vi "Query_Temp_Path.vi"(8 "error in (no error)":errorcluster, 11 "Dest_NI_MSIPath in":refnum<class "Dest_NI_MSIPath.lvclass">) -> (0 "error out":errorcluster, 3 "Dest_NI_MSIPath out":refnum<class "Dest_NI_MSIPath.lvclass">)   [LabVIEW 2020, in "Dest_NI_MSIPath.lvclass"]
uses:
  <vilib>/AppBuilder/IB_Classes/Dest_NI_MSIPath/Dest_NI_MSIPath.lvclass
  <vilib>/AppBuilder/IB_Classes/Dest_NI_MSIPath/Dest_NI_MSIPath.lvclass/Dest_NI_MSIPath.ctl
  kernel32.dll
  <vilib>/AppBuilder/IB_Classes/Destination/niLabel/niLabel.lvclass
  e:/builds/penguin/labview/branches/2020/dev/dist/vi.lib/AppBuilder/IB_Classes/Destination/niLabel/niLabel.lvclass
  e:/builds/penguin/labview/branches/2020/dev/dist/vi.lib/AppBuilder/IB_Classes/Destination/IB_Destination.lvclass
  e:/builds/penguin/labview/branches/2020/dev/dist/vi.lib/AppBuilder/IB_Classes/Dest_NI_MSIPath/Dest_NI_MSIPath.lvclass
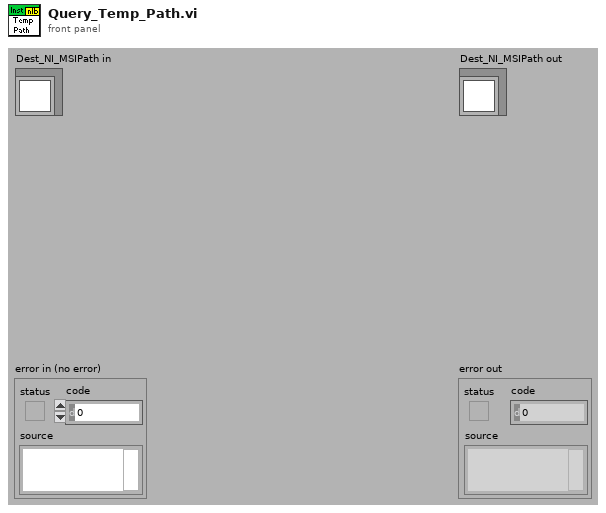
[diagram p1: front panel]
types:
  T1 = typedef "IB_Dest_niLabel.ctl" = cluster{"local path":path}
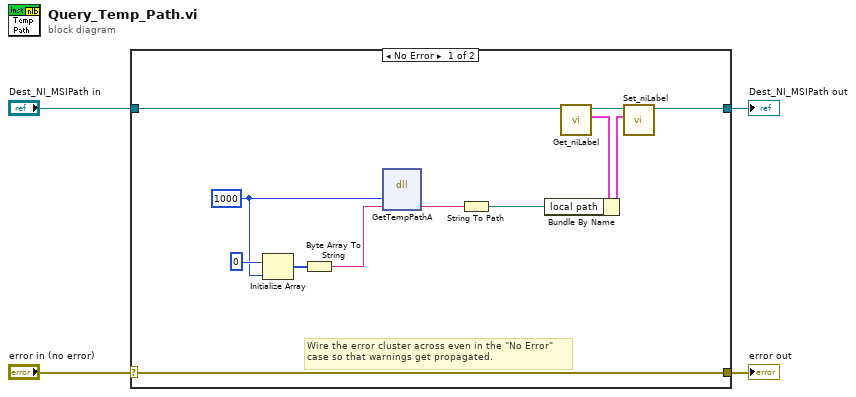
[diagram p0: block diagram]
diagram:
  n1 = case shown="No Error" "error in (no error)" {
    selector: "error in (no error)" -> [w16 w18]
    tunnel: [w16 w18] -> w3
    tunnel: [w7 w17] -> w1
    tunnel: "Dest_NI_MSIPath in" -> [w6 w17]
    frame No Error {
      w11 = u32 1000 ("dimension size")
      # "Wire the error cluster across even in the \"No Error\"\ncase so that warnings get propagated."
      n2 = Initialize Array(u8 0, w11) -> (w14:u8[])
      n3 = Byte Array To String(unsigned byte array=w14) -> (string=w13:string)
      n4 = dll-call lib="kernel32.dll" fn="GetTempPathA"("nBufferLength"=w11, "lpBuffer"=w13) -> ("lpBuffer"=w12:string)  [unwired: 5 in, 2 out]
      n5 = String To Path(string=w12) -> (path=w5:path)
      n6 = call <vilib>:"Get_niLabel.vi"("niLabel in"=w6) -> ("data"=w10:T1, "niLabel out"=w8:refnum<class "Dest_NI_MSIPath.lvclass">)  [unwired: 8 in, 1 out]
      n7 = Bundle By Name(cluster=w10, "local path"=w5) -> (w9:T1)
      n8 = call <vilib>:"Set_niLabel.vi"("data"=w9, "niLabel in"=w8) -> ("niLabel out"=w7:refnum<class "Dest_NI_MSIPath.lvclass">)  [unwired: 8 in, 1 out]
    }
    frame Error {
    }
  }
  "error out" <- w3
  "Dest_NI_MSIPath out" <- w1
